vi "test User Event Fired.vi"(8 "error in (no error)":errorcluster, 11 "TestCase in":refnum<class "Sync Tests.lvclass">) -> (0 "error out":errorcluster, 3 "TestCase out":refnum<class "Sync Tests.lvclass">)   [LabVIEW 2020, in "Sync Tests.lvclass"]
uses:
  Sync Tests.lvclass
  Sync Tests.lvclass/Sync Tests.ctl
  <vilib>/addons/_JKI Toolkits/VI Tester/TestCase.llb/TestCase.lvclass
  C:/Program Files (x86)/National Instruments/LabVIEW 2020/vi.lib/addons/_JKI Toolkits/VI Tester/TestCase.llb/TestCase.lvclass
panel:
  out "return type":i32
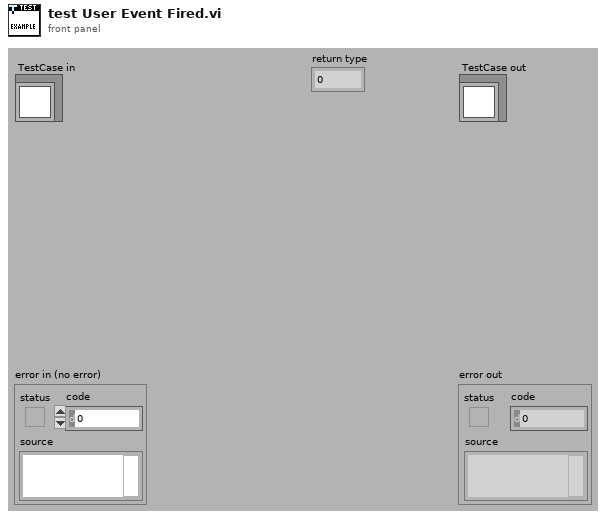
[diagram p1: front panel]
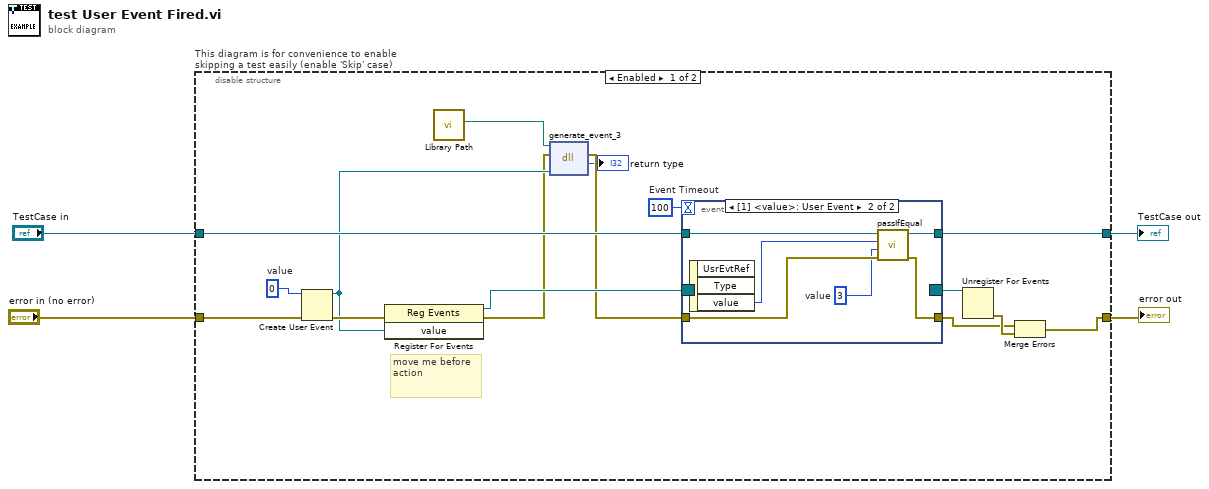
[diagram p0: block diagram]
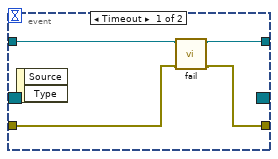
[diagram p2: hidden frame]
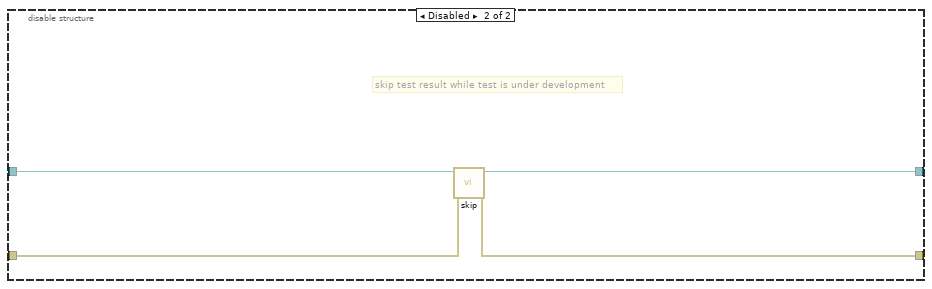
[diagram p3: hidden frame]
diagram:
  n1 = disable-structure "This diagram is for convenience to enable skipping a test easily (enable 'Skip' case)" shown="Enabled" {
    disable-tunnel: "TestCase in" -> [w12 w34]
    disable-tunnel: [w11 w32] -> w1
    disable-tunnel: [w10 w33] -> w3
    disable-tunnel: "error in (no error)" -> [w20 w31]
    frame Enabled {
      w14 = 100  # Event Timeout
      w19 = 0  # value
      # "move me before\naction"
      n2 = Create User Event(user event datatype=w19, error in=w20) -> (user event=w8:refnum<user-event>, error out=w13:errorcluster)
      n3 = register-events(error in=w13, w8) -> (reference out=w18:refnum<event-registration>, error out=w7:errorcluster)  [unwired: 1 in]
      n4 = call "Library Path.vi"() -> ("Library Path"=w9:path)  [unwired: 11 in]
      n5 = dll-call lib="C:/Users/JamesMcNally/Documents/RustInterop/Rust-LabVIEW-Interop/target/debug/labview_test_library.dll" fn="generate_event_3"(path in=w9, error in=w7, "event"=w8) -> (error out=w6:errorcluster, "return type"=→"return type":i32)  [unwired: 2 in, 1 out]
      n6 = event shown="[1] <value>: User Event" {
        selector: w18 -> [_ _]
        dyn-events: [_ _] -> w15
        timeout: w14 -> [_ _]
        tunnel: w12 -> [w24 w29]
        tunnel: [w23 w30] -> w11
        tunnel: [w21 w28] -> w16
        tunnel: w6 -> [w22 w27]
        event Timeout {
          n7 = event-data() -> ()  [unwired: 1 in, 2 out]
          n8 = call-dynamic "fail.vi"("error in (no error)"=w22, "TestCase in"=w24) -> ("error out"=w21:errorcluster, "TestCase out"=w23:refnum<class "Sync Tests.lvclass">)  [unwired: 8 in]
        }
        event User Event {
          w25 = 3  # value
          n9 = event-data() -> ("value"=w26:i32)  [unwired: 1 in, 2 out]
          n10 = call-dynamic "passIfEqual.vi"("error in (no error)"=w27, "y"=w25, "x"=w26, "TestCase in"=w29) -> ("error out"=w28:errorcluster, "TestCase out"=w30:refnum<class "Sync Tests.lvclass">)  [unwired: 6 in]
        }
      }
      n11 = Unregister For Events(event registration refnum=w15) -> (error out=w17:errorcluster)  [unwired: 1 in]
      n12 = Merge Errors(w16, w17) -> (w10:errorcluster)
    }
    frame Disabled {
      # "skip test result while test is under development"
      n13 = call <vilib>:"skip.vi"("error in (no error)"=w31, "TestCase in"=w34) -> ("error out"=w33:errorcluster, "TestCase out"=w32:refnum<class "Sync Tests.lvclass">)  [unwired: 8 in]
    }
  }
  "error out" <- w3
  "TestCase out" <- w1
